vi "CloseAll.vi"   [LabVIEW 2017, in "Communication.lvlib"]
uses:
  Communication.lvlib
  QueueRepo.Action.ctl
  MsgData.ctl
  MsgAck.ctl
  <vilib>/event_ctls.llb/usereventprio.ctl
types:
  T1 = typedef "Communication.lvlib/QueueRepo.Action.ctl" = enum16{"Add", "Get", "Destroy", "Get All", "Clear"}
  T2 = typedef "Communication.lvlib/MsgData.ctl" = cluster{"Msg":string, "Data":variant, "Ack":refnum<notifier>}
  T3 = typedef "usereventprio.ctl" = enum32{"high priority", "normal priority"}
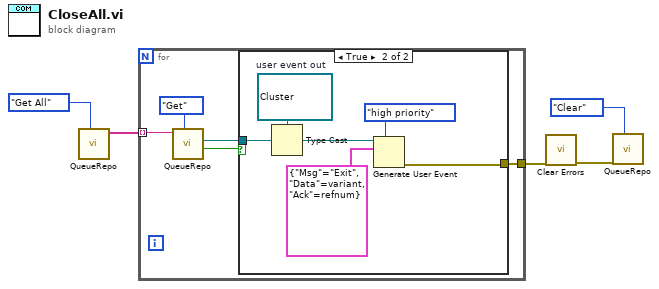
[diagram p0: block diagram]
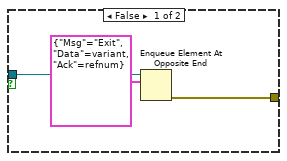
[diagram p2: hidden frame]
diagram:
  n1 = call "QueueRepo.vi"("Action"=QueueRepo.Action."Get All") -> ("Names"=w4:string[])  [unwired: 7 in, 3 out]
  n2 = for {
    tunnel: w4 -> [w10] mode=indexing
    tunnel: [w6] -> w3
    n3 = call "QueueRepo.vi"("Action"=QueueRepo.Action."Get", "Name"=w10) -> ("Event?"=w8:bool, "queue out"=w7:refnum<queue>)  [unwired: 6 in, 2 out]
    n4 = case shown="True" w8 {
      tunnel: w7 -> [w13 w19]
      tunnel: [w11 w14] -> w6
      frame False {
        n5 = Enqueue Element At Opposite End(queue=w13, element=T2 {"Msg"="Exit", "Data"=variant, "Ack"=refnum}) -> (error out=w11:errorcluster)  [unwired: 2 in, 2 out]
      }
      frame True {
        w18 = refnum<user-event> refnum  # user event out
        n6 = Type Cast(type=w18, x=w19) -> (*(type *) &x=w17:refnum<user-event>)
        n7 = Generate User Event(priority (normal)=usereventprio."high priority", user event=w17, event data cluster=T2 {"Msg"="Exit", "Data"=variant, "Ack"=refnum} ("event data")) -> (error out=w14:errorcluster)  [unwired: 1 in, 1 out]
      }
    }
  }
  n8 = call <vilib>:"Clear Errors.vi"("error in (no error)"=w3) -> ("error out"=w2:errorcluster)  [unwired: 5 in, 1 out]
  n9 = call "QueueRepo.vi"("Action"=QueueRepo.Action."Clear", "error in (no error)"=w2) -> ()  [unwired: 6 in, 4 out]
